vi "Write Panel Data Reading Event.vi"(8 "error in (no error)":errorcluster, 10 "Panel Data Reading Event":refnum<user-event>, 11 "Generic Test Stand in":refnum<class "Generic Test Stand.lvclass">) -> (0 "error out":errorcluster, 3 "Generic Test Stand out":refnum<class "Generic Test Stand.lvclass">)   [LabVIEW 2019, in "Generic Test Stand.lvclass"]
uses:
  Generic Test Stand.lvclass
  Generic Test Stand.lvclass/Generic Test Stand.ctl
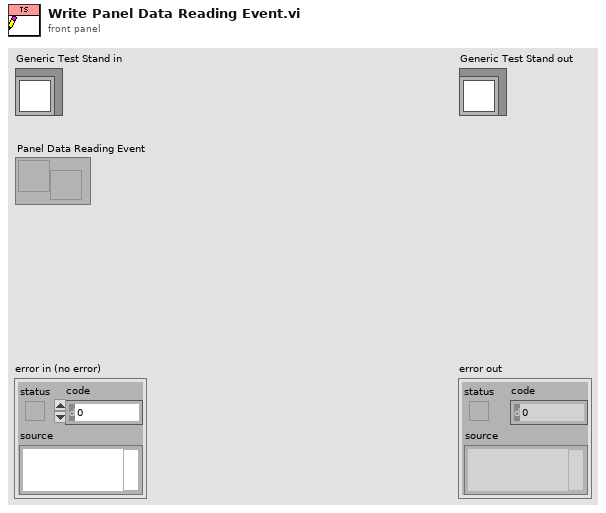
[diagram p1: front panel]
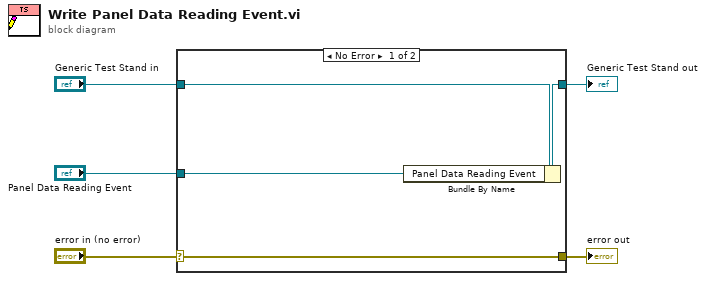
[diagram p0: block diagram]
diagram:
  n1 = case shown="No Error" "error in (no error)" {
    selector: "error in (no error)" -> [w9 w10]
    tunnel: [w9 w10] -> w4
    tunnel: [w7 w11] -> w2
    tunnel: "Generic Test Stand in" -> [w8 w11]
    tunnel: "Panel Data Reading Event" -> [w6 _]
    frame No Error {
      n2 = Bundle By Name(cluster=w8, "Panel Data Reading Event"=w6) -> (w7:refnum<class "Generic Test Stand.lvclass">)
    }
    frame Error {
    }
  }
  "error out" <- w4
  "Generic Test Stand out" <- w2
